vi "C to F (sgl).vi"(1 "C":sgl) -> (0 "F":sgl)   [LabVIEW 2012, in "Temp Converter.lvlib"]
doc: "<B>输入端子C</B>: 输入摄氏温度。\n<B>输出端子C</B>: 输出华氏温度。\n\n公式： F=C*1.8+32.\n创建者：CSXCS_366"
uses:
  Temp Converter.lvlib
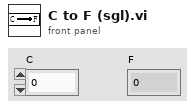
[diagram p1: front panel]
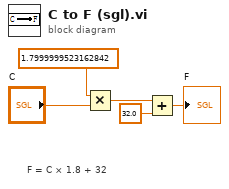
[diagram p0: block diagram]
diagram:
  # "F = C × 1.8 + 32"
  n1 = Multiply(x=sgl 1.8, y="C") -> (x*y=w2:sgl)
  n2 = Add(x=w2, y=sgl 32.0) -> (x+y=→"F":sgl)
